vi "Get Moisture Contents.vi"(6 "Related by":enum16{"Volune", "Weight"}(ring), 8 "error in (no error)":errorcluster, 9 "Gas":enum16{"SF6", "N2"}(ring), 11 "Sensor General Class in":refnum<class "Sensor General Class.lvclass">) -> (0 "error out":errorcluster, 2 "Moisture":sgl, 3 "Sensor General Class out":refnum<class "Sensor General Class.lvclass">)   [LabVIEW 2020, in "Sensor General Class.lvclass"]
uses:
  Sensor General Class.lvclass
  Data Enum.ctl
  Sensor General Class.lvclass/Sensor General Class.ctl
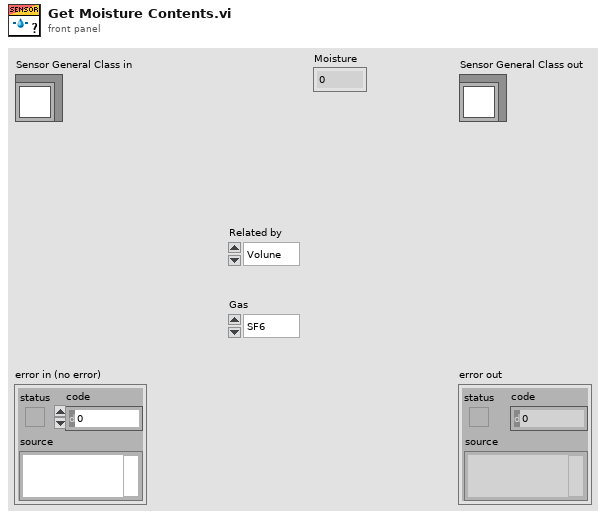
[diagram p1: front panel]
types:
  T1 = typedef "Sensor General Class.lvclass/Data Enum.ctl" = enum16{"p_bar", "p_MPa", "p_Pa", "p_kPa", "p_psi", "p_H/cm^2", "t_C", "t_K", "t_F", "rho_g/l", "rho_kg/m^3", "p20_bar", "related p20_bar", "p20_MPa", "related p20_MPa", "Tf_SF6", "Td_sf6", "tank Tf_SF6", "tank Td_SF6", "Tf_N2", "Td_N2", "tank Tf_N2", "tank Td_N2", "ppm_v SF6", "ppm_w SF6", "ppm_v N2", "ppm_w N2", "rH"}
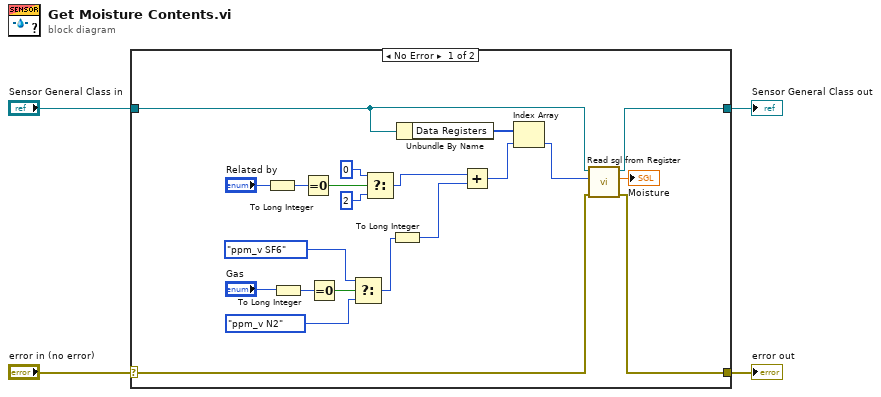
[diagram p0: block diagram]
diagram:
  n1 = case shown="No Error" "error in (no error)" {
    selector: "error in (no error)" -> [w6 w27]
    tunnel: [w7 w27] -> w3
    tunnel: [w8 w26] -> w1
    tunnel: "Sensor General Class in" -> [w9 w26]
    frame No Error {
      n2 = To Long Integer(number="Related by") -> (32bit integer=w14:i32)
      n3 = To Long Integer(number="Gas") -> (32bit integer=w20:i32)
      n4 = Equal To 0?(x=w14) -> (x = 0?=w15:bool)
      n5 = Equal To 0?(x=w20) -> (x = 0?=w19:bool)
      n6 = Select(t=Data_Enum."ppm_v SF6" ("Data Enum"), s=w19, f=Data_Enum."ppm_v N2" ("Data Enum")) -> (s? t:f=w16:T1)
      n7 = Select(t=0 ("x"), s=w15, f=2 ("x")) -> (s? t:f=w10:i32)
      n8 = To Long Integer(number=w16) -> (32bit integer=w25:i32)
      n9 = Unbundle By Name(w9) -> ("Data Registers"=w24:u16[])
      n10 = Add(x=w10, y=w25) -> (x+y=w23:i32)
      n11 = Index Array(array=w24, index=w23) -> (element=w22:u16)
      n12 = call-dynamic "Read sgl from Register.vi"("error in (no error)"=w6, "Start Register"=w22, "Sensor General Class in"=w9) -> ("error out"=w7:errorcluster, "Data"=→"Moisture":sgl, "Sensor General Class out"=w8:refnum<class "Sensor General Class.lvclass">)  [unwired: 6 in]
    }
    frame Error {
    }
  }
  "error out" <- w3
  "Sensor General Class out" <- w1
